vi "WPI_SerialPortOpen_USB.vi"(0 "Baud Rate":u32=9600, 1 "Timeout Value (ms)":u32=5000, 2 "Termination Char (0xA = '\\n' = LF)":u8=10 format="%.0x", 3 "Enable Termination Char? (T)":bool=TRUE, 5 "Data Bits":u16=8, 7 "Parity":u16(ring) items=["None", "Odd", "Even", "Mark", "Space"], 9 "Stop Bits":u16(ring)=10 items=["1.0"=10, "1.5"=15, "2.0"=20], 11 "error in (no error)":errorcluster, 12 "Flow Control":u16(ring) items=["None", "XON/XOFF", "RTS/CTS", "XON/XOFF & RTS/CTS", "DTR/DSR", "XON/XOFF & DTR/DSR"], 13 "Serial Port":T1=enum."MXP TTL") -> (4 "SerialPortRef":T2, 15 "error out":errorcluster)   [LabVIEW 2015]
doc: "Opens a reference to the serial port. You must open a reference before using any other VIs on this palette.\n\nThis software is licensed. Open the labview\\readme\\WPI Robotics Library Open Source License.txt file for more information."
uses:
  <vilib>/Rock Robotics/WPI/SerialPort/WPI_SerialPortRef.ctl
  WPI_SerialPort_USB.ctl
  <vilib>/Rock Robotics/SystemInterfaces/NetworkCommunication/NetComm_UsageReport_ResourceType.ctl
  NI WPI Serial USB.lvlib
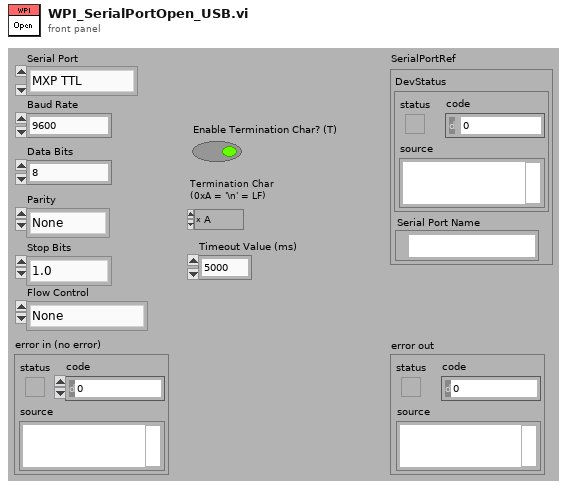
[diagram p1: front panel]
types:
  T1 = typedef "NI WPI Serial USB.lvlib/WPI_SerialPort_USB.ctl" = enum16{"Onboard RS-232", "MXP TTL", "USB"}
  T2 = typedef "WPI_SerialPortRef.ctl" = cluster{"DevStatus":errorcluster, "Serial Port Name":refnum<visa-resource-name>}
  T3 = typedef "NetComm_UsageReport_ResourceType.ctl" = enum8{"Controller", "Module", "Language", "CANPlugin", "Accelerometer", "ADXL345", "AnalogChannel", "AnalogTrigger", "AnalogTriggerOutput", "CANJaguar", "Compressor", "Counter", "Dashboard", "DigitalInput", "DigitalOutput", "DriverStationCIO", "DriverStationEIO", "DriverStationLCD", "Encoder", "GearTooth", "Gyro", "I2C", "Framework", "Jaguar", "Joystick", "Kinect", "KinectStick", "PIDController", "Preferences", "PWM", "Relay", "RobotDrive", "SerialPort", "Servo", "Solenoid", "SPI", "Task", "Ultrasonic", "Victor", "Button", "Command", "AxisCamera", "PCVideoServer", "SmartDashboard", "Talon", "HiTechnicColorSensor", "HiTechnicAccel", "HiTechnicCompass", "SRF08", "AnalogOutput", "Victor SP", "Talon SRX", "CAN Talon SRX", "ADXL362 Accel", "ADXRS450 Gyro", "Rev SPARK", "Mindsensors SD540", "Digital Filter"}
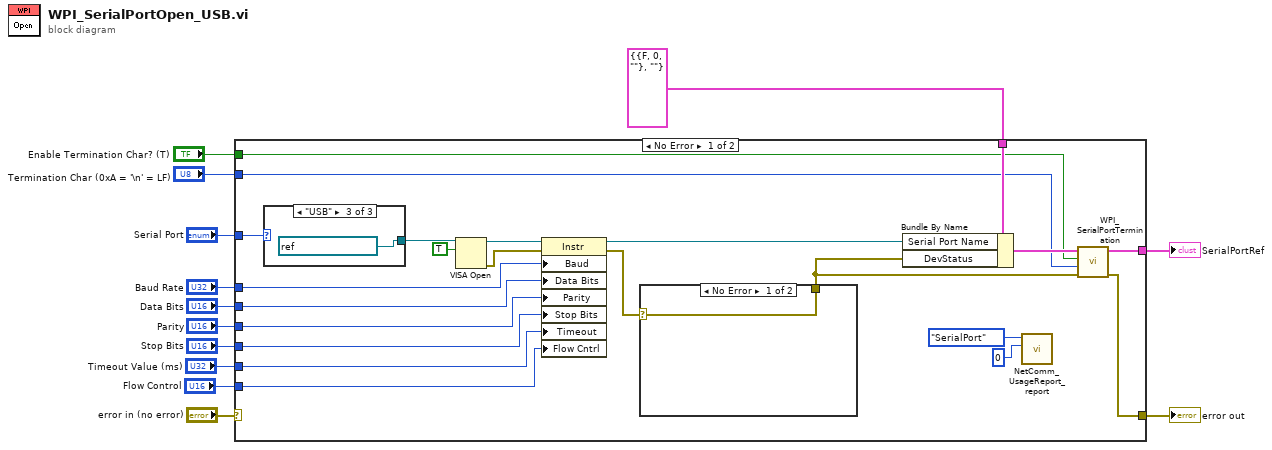
[diagram p0: block diagram]
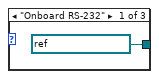
[diagram p2: hidden frame]
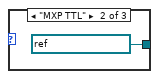
[diagram p3: hidden frame]
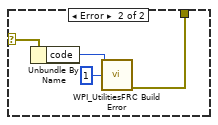
[diagram p4: hidden frame]
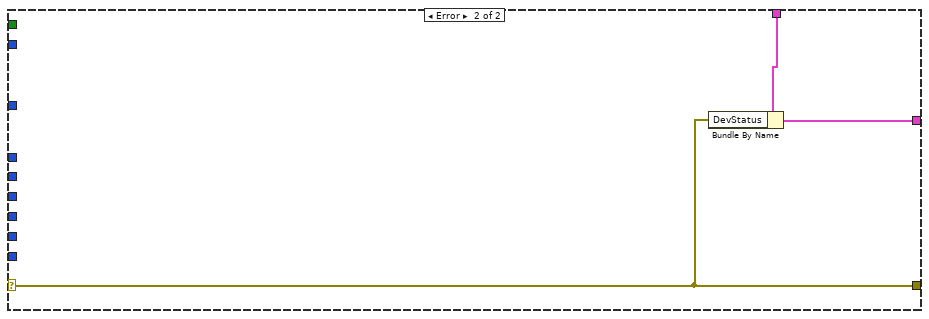
[diagram p5: hidden frame]
diagram:
  n1 = case shown="No Error" "error in (no error)" {
    selector: "error in (no error)" -> [_ w45]
    tunnel: "Baud Rate" -> [w33 _]
    tunnel: "Parity" -> [w32 _]
    tunnel: "Data Bits" -> [w31 _]
    tunnel: [w25 w46] -> w10
    tunnel: "Stop Bits" -> [w21 _]
    tunnel: [w26 w45] -> w7
    tunnel: T2 {"DevStatus"={"status"=FALSE, "code"=0, "source"=""}, "Serial Port Name"=""} ("SerialPortRef") -> [w29 w44]
    tunnel: "Enable Termination Char? (T)" -> [w23 _]
    tunnel: "Termination Char (0xA = '\\n' = LF)" -> [w24 _]
    tunnel: "Timeout Value (ms)" -> [w22 _]
    tunnel: "Flow Control" -> [w20 _]
    tunnel: "Serial Port" -> [w15 _]
    frame No Error {
      n2 = case shown="\"USB\"" w15 {
        tunnel: [refnum<visa-resource-name> "ASRL1::INSTR" ("VISA resource name") refnum<visa-resource-name> "ASRL2::INSTR" ("VISA resource name") refnum<visa-resource-name> "ASRL3::INSTR" ("VISA resource name")] -> w14
        frame "Onboard RS-232" {
        }
        frame "MXP TTL" {
        }
        frame "USB" {
        }
      }
      n3 = VISA Open(duplicate session (F)=TRUE, VISA resource name=w14) -> (VISA resource name=w35:refnum<visa-resource-name>, error out=w34:errorcluster)  [unwired: 1 in, 2 out]
      n4 = property class="Instr"(reference=w35, error in=w34, "Baud"=w33, "Data Bits"=w31, "Parity"=w32, "Stop Bits"=w21, "Timeout"=w22, "Flow Cntrl"=w20) -> (reference out=w30:refnum<visa-resource-name>, error out=w19:errorcluster)
      n5 = case shown="No Error" w19 {
        selector: w19 -> [w39 w41]
        tunnel: [w39 w40] -> w18
        frame No Error {
        }
        frame Error {
          n6 = Unbundle By Name(w41) -> ("code"=w43:i32)
          n7 = call <vilib>:"WPI_UtilitiesFRC Build Error.vi"("error code"=w43, "chain levels to remove (1)"=1) -> ("error out"=w40:errorcluster)  [unwired: 3 in, 10 out]
        }
      }
      n8 = Bundle By Name(cluster=w29, "Serial Port Name"=w30, "DevStatus"=w18) -> (w27:T2)
      n9 = call <vilib>:"NetComm_UsageReport_report.vi"("Instance Number"=u8 0, "Resource Type"=NetComm_UsageReport_ResourceType."SerialPort") -> ()  [unwired: 10 in]
      n10 = call <vilib>:"WPI_SerialPortTermination.vi"("error in (no error)"=w18, "Termination Char (0xA = '\\n' = LF)"=w24, "Enable? (T)"=w23, "SerialPortRef"=w27) -> ("error out"=w26:errorcluster, "SerialPortRef"=w25:T2)  [unwired: 6 out]
    }
    frame Error {
      n11 = Bundle By Name(cluster=w44, "DevStatus"=w45) -> (w46:T2)
    }
  }
  "error out" <- w7
  "SerialPortRef" <- w10
